vi "global_queue.vi"() -> ()   [LabVIEW 2011]
panel:
  in  "queue out":refnum<queue>
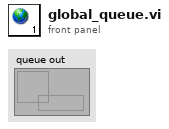
[diagram p1: front panel]
diagram:
